vi "Read HH Status.vi"(8 "error in (no error)":errorcluster, 11 "DCM-DSI-HW in":refnum<class "DCM-DSI.lvclass">) -> (0 "error out":errorcluster, 2 "HH Status":T1[](array[typedef]) {"Current [A]" format="%#_6p"; "On Avg [A]" format="%#_6p"; "Period Avg [A]" format="%#_6p"; "Period Max [A]" format="%#_6p"; "Period Min [A]" format="%#_6p"}, 3 "DCM-DSI-HW out":refnum<class "DCM-DSI.lvclass">)   [LabVIEW 2016, in "DCM-DSI.lvclass"]
uses:
  DCM-DSI.lvclass
  <vilib>/Powertrain Controls/Device Drivers/DCM/HH/RT/Status.ctl
  DCM-DSI.lvclass/DCM-DSI.ctl
  <vilib>/Powertrain Controls/Device Drivers/DCM/HH/RT/DCM - RT - HH.lvlib
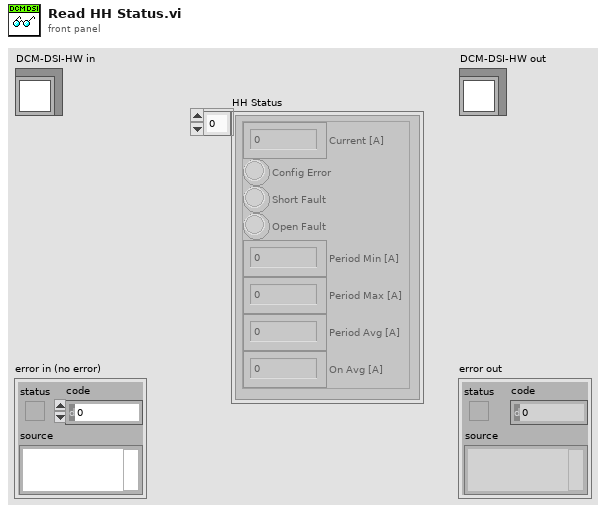
[diagram p1: front panel]
types:
  T1 = typedef "DCM - RT - HH.lvlib/Status.ctl" = cluster{"Current [A]":sgl, "Config Error":bool, "Short Fault":bool, "Open Fault":bool, "Period Min [A]":sgl, "Period Max [A]":sgl, "Period Avg [A]":sgl, "On Avg [A]":sgl}
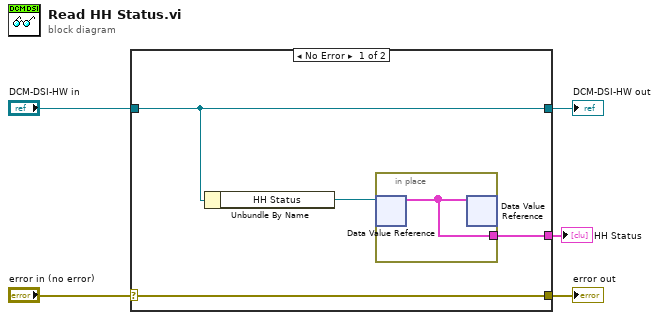
[diagram p0: block diagram]
diagram:
  n1 = case shown="No Error" "error in (no error)" {
    selector: "error in (no error)" -> [w9 w12]
    tunnel: [w9 w12] -> w4
    tunnel: [w7 w11] -> w2
    tunnel: "DCM-DSI-HW in" -> [w7 w11]
    tunnel: [w6 _] -> w1
    frame No Error {
      n2 = Unbundle By Name(w7) -> ("HH Status"=w8:refnum<data-value>)
      n3 = in-place {
        in-place-border: [w10] -> w6
        n4 = in-place-dvr #1(w8) -> (w10:T1[])  [unwired: 1 out]
        n5 = in-place-dvr #1(w10) -> ()  [unwired: 2 out]
      }
    }
    frame Error {
    }
  }
  "error out" <- w4
  "DCM-DSI-HW out" <- w2
  "HH Status" <- w1
